vi "Map_GetMaps.vi"(11 "Map Path":path) -> (2 "Map Plane 1":u8[](array[numeric]), 3 "Map Plane 0":u8[](array[numeric]))   [LabVIEW 2020]
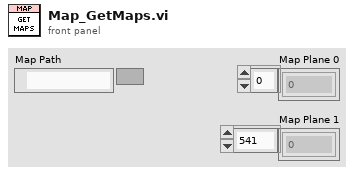
[diagram p1: front panel]
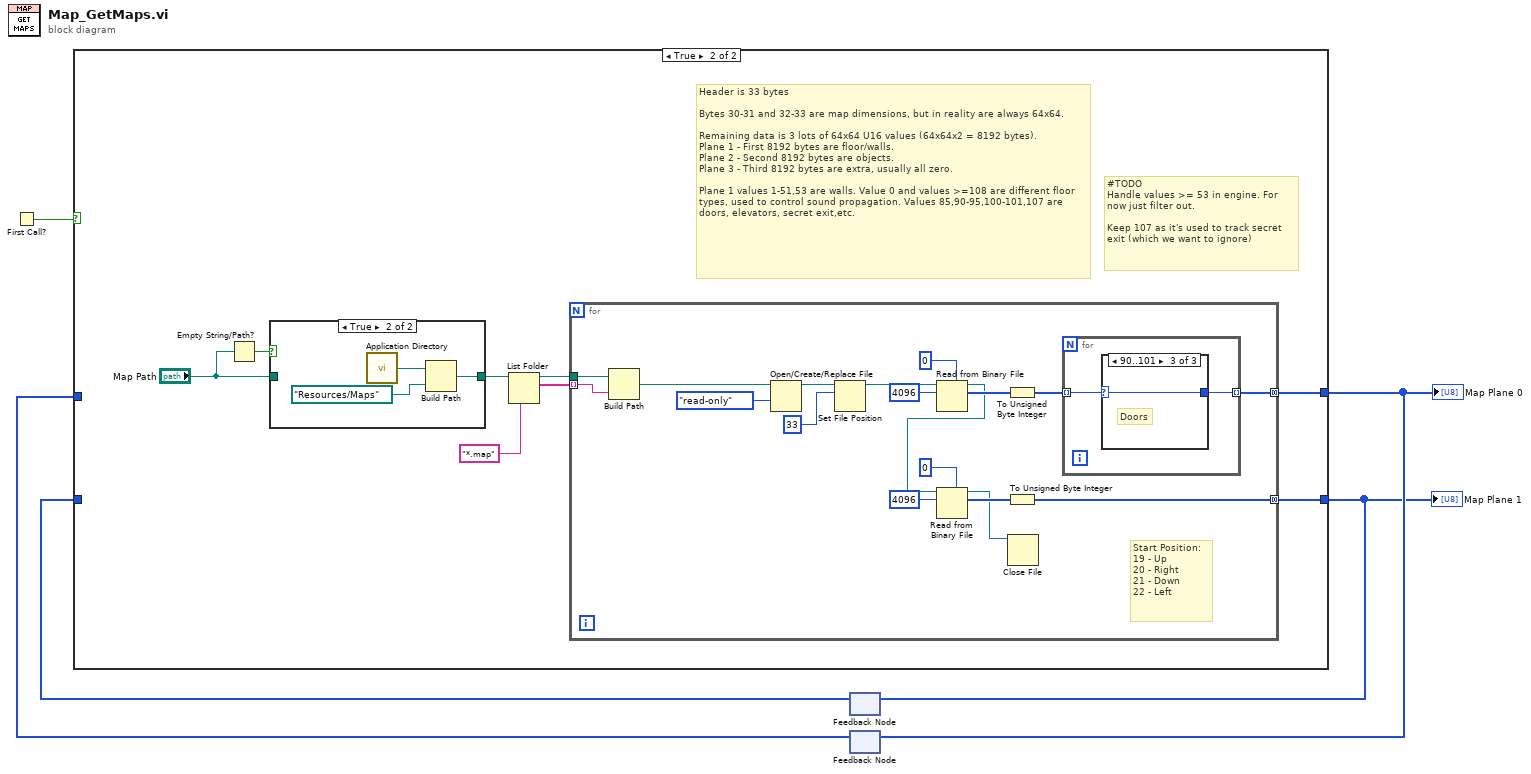
[diagram p0: block diagram]
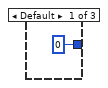
[diagram p3: hidden frame]
diagram:
  n1 = First Call?() -> (First Call?: T/F=w5:bool)
  n2 = feedback #1() -> (w2:u8[])  [unwired: 1 in]
  n3 = feedback #2() -> (w4:u8[])  [unwired: 1 in]
  n4 = case shown="True" w5 {
    tunnel: [w7 w15] -> w3
    tunnel: w4 -> [w7 _]
    tunnel: [w6 w14] -> w1
    tunnel: w2 -> [w6 _]
    frame False {
    }
    frame True {
      # "#TODO\nHandle values >= 53 in engine. For now just filter out.\n\nKeep 107 as it's used to track secret exit (which we want to ignore)"
      # "Header is 33 bytes\n\nBytes 30-31 and 32-33 are map dimensions, but in reality are always 64x64.\n\nRemaining data is 3 lots of 64x64 U16 values (64x64x2 = 8192 bytes).\nPlane 1 - First 8192 bytes are floor/walls.\nPlane 2 - Second 8192 bytes are objects.\nPlane 3 - Third 8192 bytes are extra, usually all zero.\n\nPlane 1 values 1-51,53 are walls. Value 0 and values >=108 are different floor types, used to control sound propagation. Values 85,90-95,100-101,107 are doors, elevators, secret exit,etc."
      n5 = Empty String/Path?(string/path="Map Path") -> (empty?=w9:bool)
      n6 = case shown="True" w9 {
        tunnel: [w39 w40] -> w13
        tunnel: "Map Path" -> [w39 _]
        frame False {
        }
        frame True {
          n7 = call <vilib>:"Application Directory.vi"() -> ("Application Directory"=w42:path)
          n8 = Build Path(base path=w42, name or relative path=path "Resources/Maps") -> (appended path=w40:path)
        }
      }
      n9 = List Folder(path=w13, pattern="*.map") -> (path out=w10:path, filenames=w11:string[])  [unwired: 2 in, 2 out]
      n10 = for {
        tunnel: [w25] -> w15 mode=concatenating
        tunnel: [w20] -> w14 mode=concatenating
        tunnel: w11 -> [w17] mode=indexing
        tunnel: w10 -> [w18]
        # "Start Position:\n19 - Up\n20 - Right\n21 - Down\n22 - Left"
        n11 = Build Path(base path=w18, name or relative path=w17) -> (appended path=w16:path)
        n12 = Open/Create/Replace File(file path (use dialog)=w16, access (0:read/write)=enum16{"read/write", "read-only", "write-only"}."read-only") -> (refnum out=w32:refnum<file>)  [unwired: 4 in, 2 out]
        n13 = Set File Position(offset (in bytes) (0)=i64 33, refnum=w32) -> (refnum out=w30:refnum<file>)  [unwired: 2 in, 1 out]
        n14 = Read from Binary File(5:u16 0 ("count (1)"), 10:4096 ("count (1)"), 11:w30) -> (2:w26:u16[], 3:w22:refnum<file>)  [unwired: 3 in, 2 out]
        n15 = Read from Binary File(5:u16 0 ("count (1)"), 10:4096 ("count (1)"), 11:w22) -> (2:w21:u16[], 3:w19:refnum<file>)  [unwired: 3 in, 2 out]
        n16 = To Unsigned Byte Integer(number=w26) -> (unsigned 8bit integer=w27:u8[])
        n17 = To Unsigned Byte Integer(number=w21) -> (unsigned 8bit integer=w20:u8[])
        n18 = Close File(refnum=w19) -> ()  [unwired: 1 in, 2 out]
        n19 = for {
          tunnel: w27 -> [w35] mode=indexing
          tunnel: [w34] -> w25 mode=indexing
          n20 = case shown="90..101" w35 {
            selector: w35 -> [_ w37 w38]
            tunnel: [u8 0 ("count (1)") w37 w38] -> w34
            frame Default {
            }
            frame 0..52, 107 {
            }
            frame 90..101 {
              # "Doors"
            }
          }
        }
      }
    }
  }
  "Map Plane 0" <- w3
  "Map Plane 1" <- w1
  n21 = feedback-in #1(w1) -> ()
  n22 = feedback-in #2(w3) -> ()
